vi "GPIB Simple Interface.vi"(8 "Error In":errorcluster) -> (0 "Error Out":errorcluster)   [LabVIEW 2014]
panel:
  in  "GPIB Address":string
  in  "Send":bool
  in  "Write String":string
  out "Read String":string
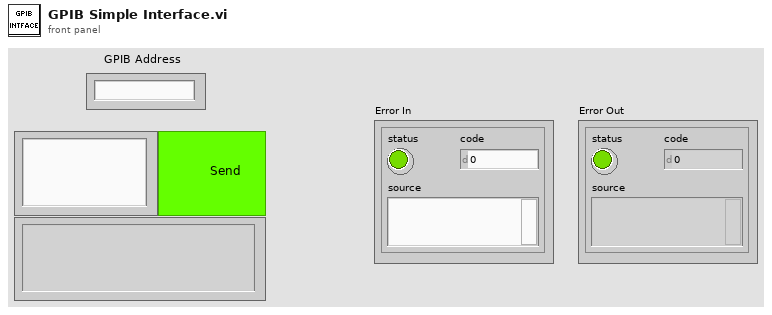
[diagram p1: front panel]
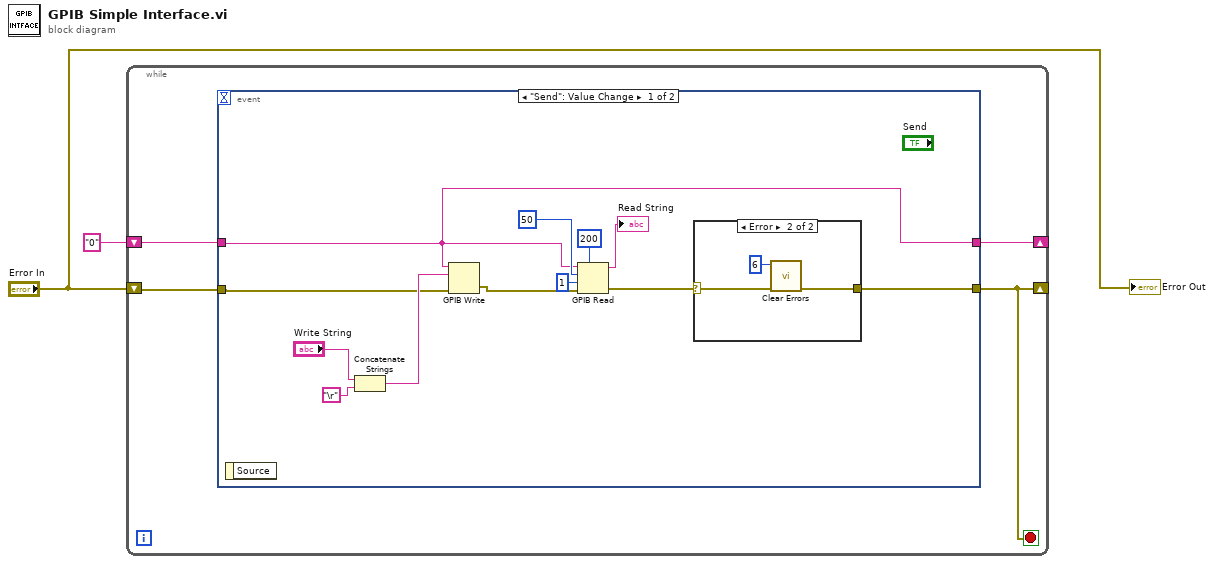
[diagram p0: block diagram]
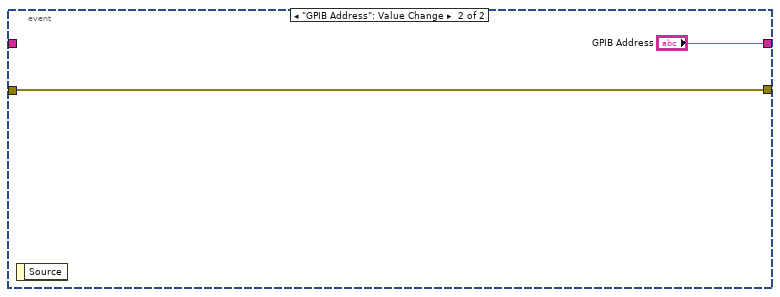
[diagram p3: hidden frame]
diagram:
  n1 = while {
    shift-right: [w4] -> _
    shift-left: "Error In" -> [w5]
    shift-right: [w3] -> _
    shift-left: "0" ("GPIB Address") -> [w6]
    stop <- w4 stop-if-true
    n2 = event shown="[0] \"Send\": Value Change" {
      selector: _ -> [_ _]
      dyn-events: _ -> [_ _]
      timeout: _ -> [_ _]
      tunnel: w6 -> [w7 _]
      tunnel: w5 -> [w9 w23]
      tunnel: [w8 w23] -> w4
      tunnel: [w7 "GPIB Address"] -> w3
      event "Send": Value Change {
        n3 = event-data() -> ()  [unwired: 1 in, 1 out]
        n4 = Concatenate Strings("Write String", "\r") -> (w15:string)
        n5 = GPIB Write(0:w7, 1:w15, 3:w9) -> (6:w16:errorcluster)  [unwired: 2 in, 1 out]
        n6 = GPIB Read(0:w7, 1:50 ("byte count"), 2:i16 1 ("mode (0)"), 3:w16, 4:200 ("timeout ms (488.2 global)")) -> (5:→"Read String":string, 7:w10:errorcluster)  [unwired: 1 out]
        n7 = case shown="Error" w10 {
          selector: w10 -> [w19 w21]
          tunnel: [w19 w20] -> w8
          frame No Error {
          }
          frame Error {
            n8 = call <vilib>:"Clear Errors.vi"("error in (no error)"=w21, "specific error code to clear (0: all)"=6) -> ("error out"=w20:errorcluster)  [unwired: 4 in, 1 out]
          }
        }
      }
      event "GPIB Address": Value Change {
        n9 = event-data() -> ()  [unwired: 1 in, 1 out]
      }
    }
  }
  "Error Out" <- "Error In"
